vi "subGetSourceItemNames.vi"(11 "Refnum in":refnum<k20>) -> (3 "Names":string[](array[string]))   [LabVIEW 2020, in "SolutionBuilder.lvlib"]
uses:
  SolutionBuilder.lvlib
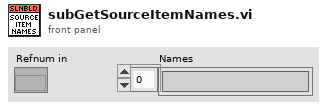
[diagram p1: front panel]
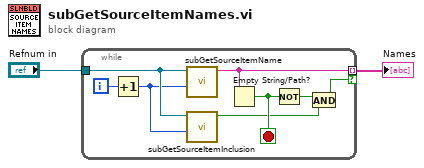
[diagram p0: block diagram]
diagram:
  n1 = while {
    tunnel: [w9] -> w2 mode=indexing if=w3
    tunnel: "Refnum in" -> [w7]
    i -> [w10]
    stop <- w8 stop-if-true
    n2 = Increment(x=w10) -> (x+1=w6:i32)
    n3 = call "subGetSourceItemName.vi"("index (1)"=w6, "Refnum in"=w7) -> ("source name"=w9:string)  [unwired: 9 in]
    n4 = call "subGetSourceItemInclusion.vi"("index (1)"=w6, "Refnum in"=w7) -> ("Include?"=w4:bool)  [unwired: 9 in]
    n5 = Empty String/Path?(string/path=w9) -> (empty?=w8:bool)
    n6 = Not(x=w8) -> (.not. x?=w5:bool)
    n7 = And(x=w5, y=w4) -> (x .and. y?=w3:bool)
  }
  "Names" <- w2
